vi "Sort Packages.vi"(11 "Packages":refnum<class "Package.lvclass">[](array[class])) -> (3 "Sorted Packages":refnum<class "Package.lvclass">[](array[class]))   [LabVIEW 2020, in "WSsupport.lvlib"]
uses:
  WSsupport.lvlib
  Packages/Package_class/Package.lvclass
  Packages/Package_class/Package.lvclass/Package.ctl
  Packages/Package_class/Read DisplayName.vi
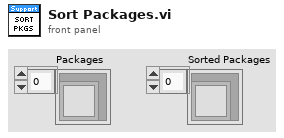
[diagram p1: front panel]
types:
  T1 = cluster{string, "Packages.lvlib:Package":refnum<class "Package.lvclass">}
  T2 = cluster{string, "Packages.lvlib:Package":refnum<class "Package.lvclass">}[]
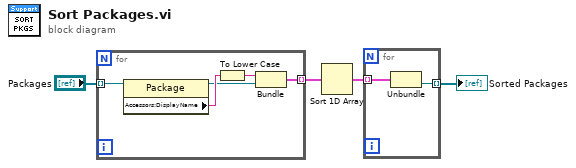
[diagram p0: block diagram]
diagram:
  n1 = for {
    tunnel: "Packages" -> [w9] mode=indexing
    tunnel: [w5] -> w3 mode=indexing
    n2 = property class="Package"(reference=w9) -> (reference out=w7:refnum<class "Package.lvclass">, "Accessors:DisplayName"=w8:string)  [unwired: 1 in, 1 out]
    n3 = To Lower Case(string=w8) -> (all lower case string=w6:string)
    n4 = Bundle(w6, "Packages.lvlib:Package"=w7) -> (w5:T1)  [unwired: 1 in]
  }
  n5 = Sort 1D Array(array=w3) -> (sorted array=w2:T2)
  n6 = for {
    tunnel: w2 -> [w11] mode=indexing
    tunnel: [w10] -> w1 mode=indexing
    n7 = Unbundle(w11) -> ("Packages.lvlib:Package"=w10:refnum<class "Package.lvclass">)  [unwired: 1 out]
  }
  "Sorted Packages" <- w1
